vi "-8730 Attribute not found--error.vi"(8 "error in":errorcluster, 11 "Attribute":string) -> (0 "error out":errorcluster)   [LabVIEW 2019, in "Config from JSON.lvclass"]
uses:
  Config from JSON.lvclass
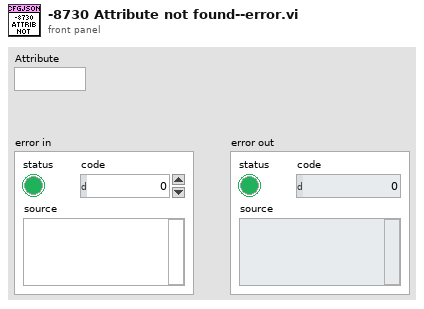
[diagram p1: front panel]
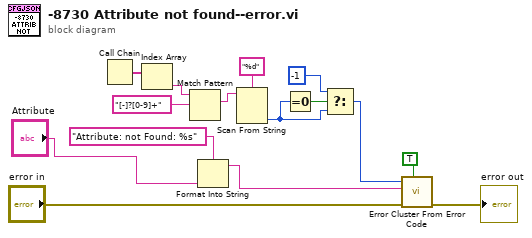
[diagram p0: block diagram]
diagram:
  n1 = Call Chain() -> (call chain=w2:string[])
  n2 = Index Array(array=w2) -> (element=w7:string)  [unwired: 1 in]
  n3 = Match Pattern(string=w7, regular expression="[-]?[0-9]+") -> (match substring=w8:string)  [unwired: 1 in, 3 out]
  n4 = Format Into String(format string="Attribute: not Found: %s" ("error message (\"\")"), "Attribute") -> (resulting string=w13:string)  [unwired: 2 in, 1 out]
  n5 = Scan From String(format string="%d", input string=w8) -> (output 1=w4:i32)  [unwired: 3 in, 3 out]
  n6 = Equal To 0?(x=w4) -> (x = 0?=w5:bool)
  n7 = Select(t=-1, s=w5, f=w4) -> (s? t:f=w1:i32)
  n8 = call <vilib>:"Error Cluster From Error Code.vi"("show call chain? (False)"=TRUE, "error in (no error)"="error in", "error message (\"\")"=w13, "error code (0)"=w1) -> ("error out"=→"error out":errorcluster)  [unwired: 5 in]
